vi "Set Named Range.vi"(7 "Sheet Name":string, 8 "error in":errorcluster, 9 "Cell Range":string="A1:B1", 10 "Named Range Identifier":string, 11 "SpreadsheetDoc in":refnum<k24>) -> (0 "error out":errorcluster, 3 "SpreadsheetDoc out":refnum<k24>)   [LabVIEW 2021, in "Open Xml.lvlib"]
uses:
  Open Xml.lvlib
  D:/git/Open-Xml-LabVIEW/dll/DocumentFormat.OpenXml.dll
  dll/DocumentFormat.OpenXml.dll
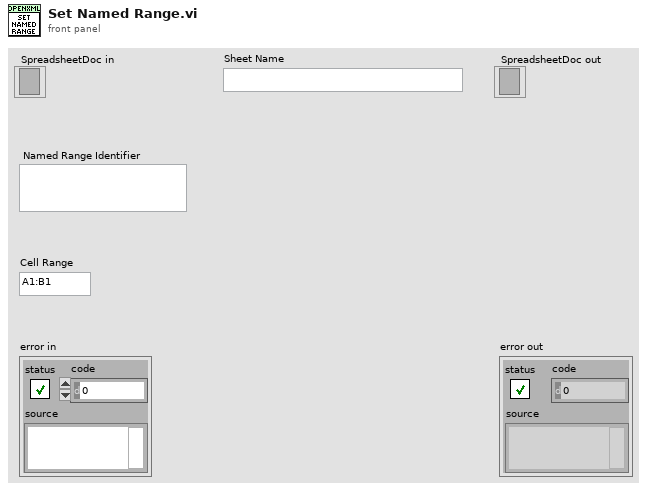
[diagram p1: front panel]
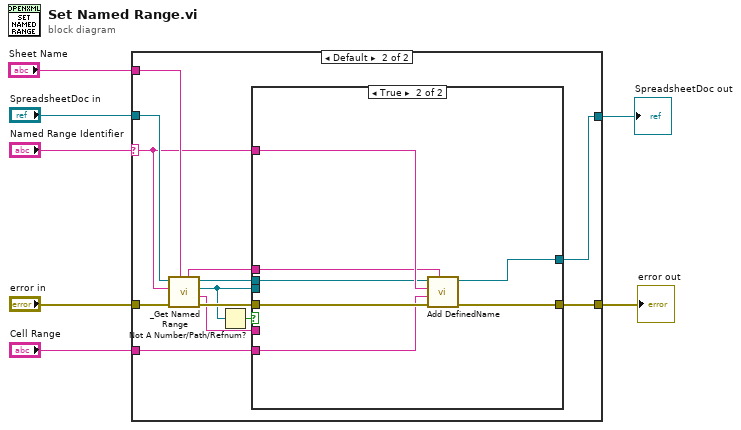
[diagram p0: block diagram]
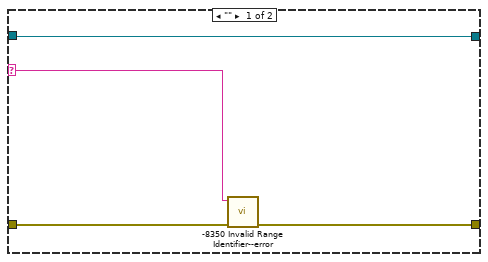
[diagram p2: hidden frame]
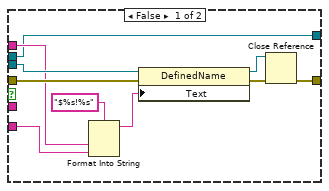
[diagram p3: hidden frame]
diagram:
  n1 = case shown="Default" "Named Range Identifier" {
    selector: "Named Range Identifier" -> [w9 w16]
    tunnel: "error in" -> [w11 w24]
    tunnel: [w10 w21] -> w6
    tunnel: "SpreadsheetDoc in" -> [w8 w22]
    tunnel: [w8 w14] -> w4
    tunnel: "Sheet Name" -> [_ w20]
    tunnel: "Cell Range" -> [_ w15]
    frame "" {
      n2 = call "-8350 Invalid Range Identifier--error.vi"("error in"=w11, "Argument"=w9) -> ("error out"=w10:errorcluster)  [unwired: 9 in]
    }
    frame Default {
      n3 = call "_Get Named Range.vi"("Sheet Name"=w20, "error in"=w24, "Range Identifier"=w16, "SpreadsheetDoc in"=w22) -> ("error out"=w23:errorcluster, "Range"=w13:string, "DefinedName"=w12:refnum<k24>, "SpreadsheetDoc out"=w18:refnum<k24>, "Sheet Name"=w19:string)  [unwired: 3 in]
      n4 = Not A Number/Path/Refnum?(number/path/refnum=w12) -> (NaN/Path/Refnum?=w17:bool)
      n5 = case shown="True" w17 {
        tunnel: w23 -> [w34 w41]
        tunnel: w18 -> [w25 w37]
        tunnel: [w27 w40] -> w21
        tunnel: w19 -> [w29 w36]
        tunnel: w16 -> [_ w39]
        tunnel: w15 -> [w28 w38]
        tunnel: [w25 w35] -> w14
        tunnel: w13 -> [_ _]
        tunnel: w12 -> [w32 _]
        frame False {
          n6 = Format Into String(format string="$%s!%s", w29, w28) -> (resulting string=w31:string)  [unwired: 2 in, 1 out]
          n7 = property class="DefinedName"(reference=w32, error in=w34, "Text"=w31) -> (reference out=w26:refnum<k24>, error out=w33:errorcluster)
          n8 = Close Reference(reference=w26, error in (no error)=w33) -> (error out=w27:errorcluster)
        }
        frame True {
          n9 = call "Add DefinedName.vi"("Sheet Name"=w36, "error in"=w41, "Cell Range"=w38, "Identifier"=w39, "SpreadsheetDoc in"=w37) -> ("error out"=w40:errorcluster, "SpreadsheetDoc out"=w35:refnum<k24>)  [unwired: 5 in]
        }
      }
    }
  }
  "error out" <- w6
  "SpreadsheetDoc out" <- w4
